vi "Check if Initialized.vi"(8 "error in (no error)":errorcluster, 11 "Device in":refnum<class "Device.lvclass">) -> (0 "error out":errorcluster, 2 "Initialized":bool, 3 "Device out":refnum<class "Device.lvclass">)   [LabVIEW 2015, in "Device.lvlib" / "Device.lvclass"]
uses:
  Device.lvclass
  <vilib>/ErrorRing/Error Ring.xnode
  <vilib>/Utility/error.llb/Error Cluster From Error Code.vi
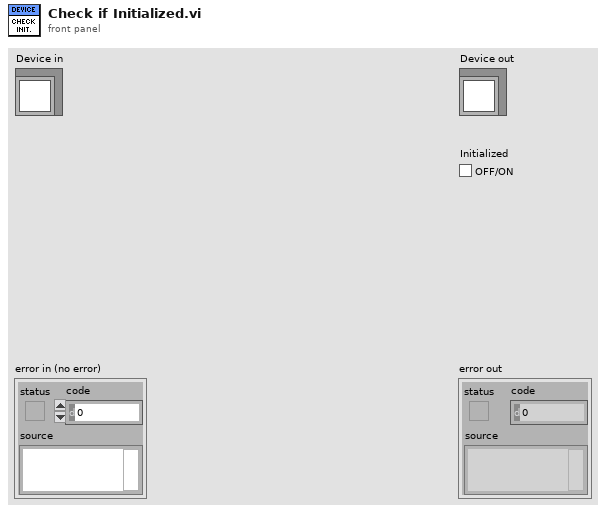
[diagram p1: front panel]
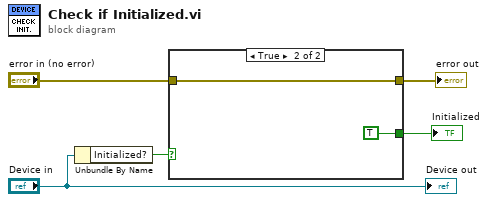
[diagram p0: block diagram]
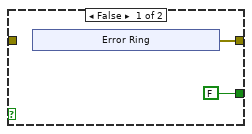
[diagram p2: hidden frame]
diagram:
  n1 = Unbundle By Name("Device in") -> ("Initialized?"=w4:bool)
  n2 = case shown="True" w4 {
    tunnel: "error in (no error)" -> [_ w14]
    tunnel: [w7 w14] -> w2
    tunnel: [FALSE TRUE] -> w1
    frame False {
      n3 = xnode "Error Ring"() -> ("error out"=w7:errorcluster)
    }
    frame True {
    }
  }
  "error out" <- w2
  "Initialized" <- w1
  "Device out" <- "Device in"
